vi "SubVI_Interpolate_Impedances.vi"(8 "error in (no error)":errorcluster, 9 "Resampling rate":dbl, 10 "Interpolant Size":dbl, 11 "Raw Impedances In":T1) -> (0 "error out":errorcluster, 3 "Interpolated Impedances Out":T2)   [LabVIEW 2020]
uses:
  <extravilib>/ChannelInstances/Stream-a[.](dbl)/)Channel.ctl
  <extravilib>/ChannelInstances/Lossy Stream-a[.](dbl)/)Channel.ctl
  <extravilib>/ChannelInstances/Lossy Stream-a[.](dbl)/EndpointRead.vi
  <extravilib>/ChannelInstances/Stream-a[.](dbl)/Endpoint.vi
  Global 1.vi
  <extravilib>/ChannelInstances/Lossy Stream-a[.](dbl)/)Channel.vi
  <resource>/ChannelSupport/_ChannelSupport/WaitIfNeeded.vi
  <extravilib>/ChannelInstances/Stream-a[.](dbl)/)Channel.vi
  <vilib>/ptbypt/NI_PtbyPt.lvlib
  <extravilib>/ChannelInstances/Stream-a[.](dbl).lvlib
  <extravilib>/ChannelInstances/Lossy Stream-a[.](dbl).lvlib
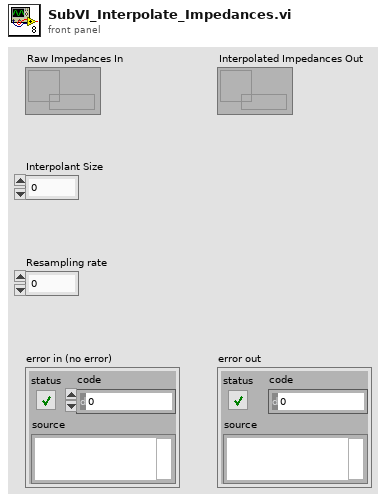
[diagram p1: front panel]
types:
  T1 = typedef "Lossy Stream-a[.](dbl).lvlib/)Channel.ctl" = refnum<queue>
  T2 = typedef "Stream-a[.](dbl).lvlib/)Channel.ctl" = refnum<queue>
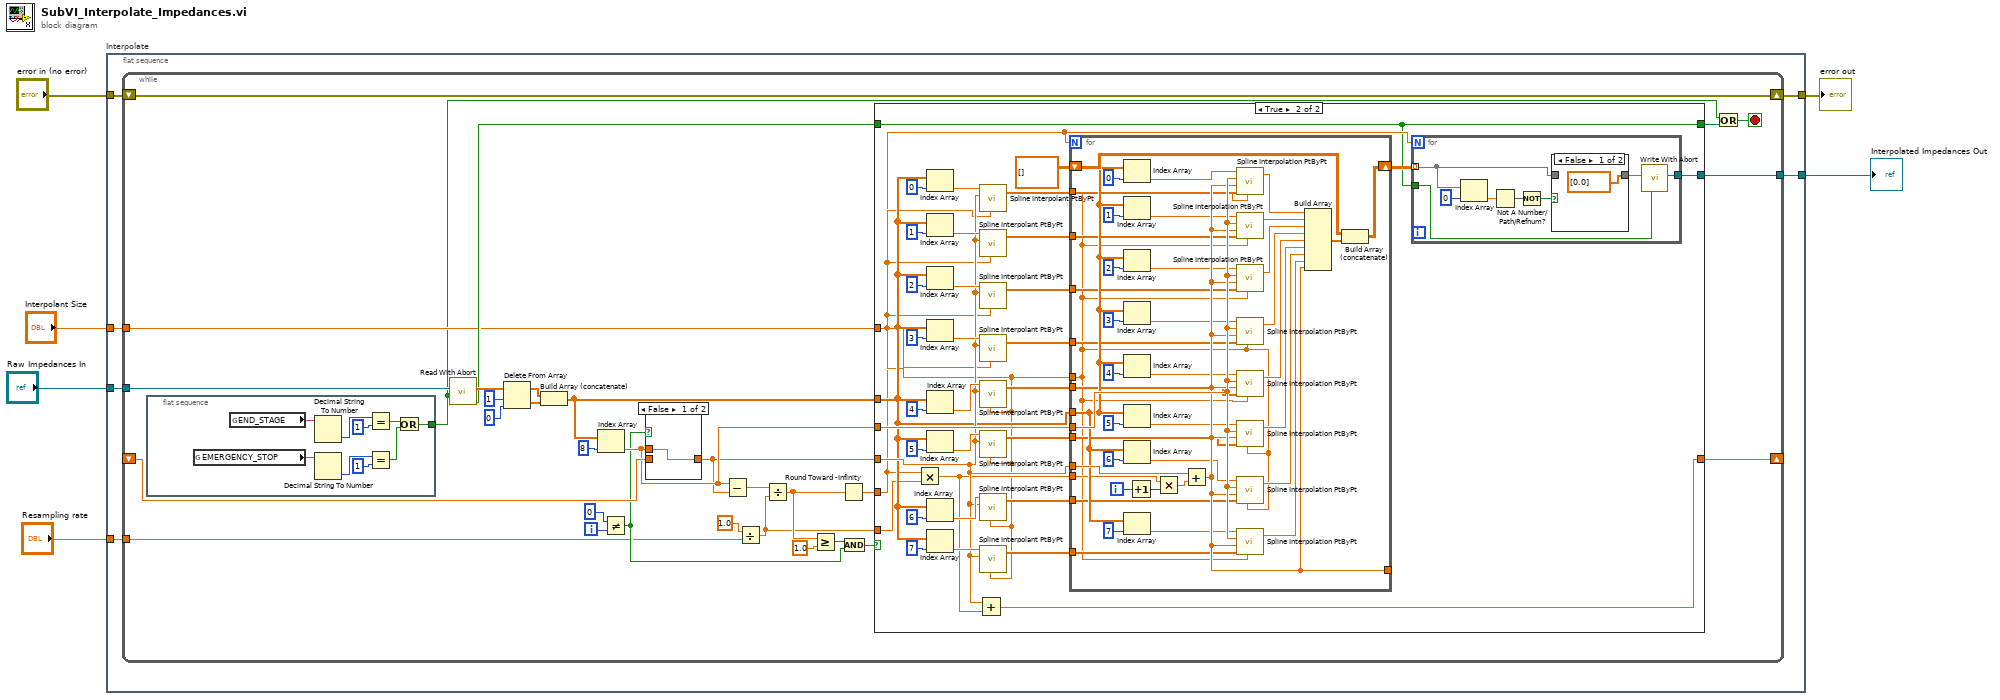
[diagram p0: block diagram]
diagram:
  n1 = flat-sequence "Interpolate" {
    tunnel: "Raw Impedances In" -> [w12]
    tunnel: [w11] -> w2
    tunnel: [w10] -> w3
    tunnel: "Interpolant Size" -> [w9]
    tunnel: "error in (no error)" -> [w8]
    tunnel: "Resampling rate" -> [w7]
    frame #0 {
      n2 = while {
        tunnel: w12 -> [w43]
        shift-right: [w26] -> _
        shift-left: _ -> [w31]
        shift-right: [w23] -> w11
        shift-left: w8 -> [w23]
        tunnel: w9 -> [w18]
        tunnel: [w17] -> w10
        tunnel: w7 -> [w16]
        i -> [w19]
        stop <- w21 stop-if-true
        n3 = flat-sequence {
          tunnel: [w44] -> w13
          frame #0 {
            n4 = global read "Global 1.vi" "EMERGENCY_STOP"() -> (w47:string)
            n5 = global read "Global 1.vi" "END_STAGE"() -> (w52:string)
            n6 = Decimal String To Number(string=w52) -> (number=w51:i32)  [unwired: 2 in, 1 out]
            n7 = Decimal String To Number(string=w47) -> (number=w49:i32)  [unwired: 2 in, 1 out]
            n8 = Equal?(x=w51, y=1) -> (x = y?=w45:bool)
            n9 = Equal?(x=w49, y=1) -> (x = y?=w46:bool)
            n10 = Or(x=w45, y=w46) -> (x .or. y?=w44:bool)
          }
        }
        n11 = call <extravilib>:"Read With Abort.vi"("abort"=w13, "channel"=w43) -> ("element"=w42:dbl[], "aborted?"=w27:bool)  [unwired: 3 in, 5 out]
        n12 = Delete From Array(array=w42, length=1, index=0) -> (deleted portion=w39:dbl[], array with subset deleted=w20:dbl[])
        n13 = Build Array (concatenate)(w20, w39) -> (w24:dbl[])
        n14 = Index Array(array=w24, index=8 ("disabled index (col)")) -> (element=w30:dbl)
        n15 = Not Equal?(x=0, y=w19) -> (x != y?=w25:bool)
        n16 = case shown="False" w25 {
          tunnel: w31 -> [_ w54]
          tunnel: [w53 w54] -> w28
          tunnel: w30 -> [w53 _]
          frame False {
          }
          frame True {
          }
        }
        n17 = Subtract(x=w30, y=w28) -> (x-y=w35:dbl)
        n18 = Divide(x=1.0 ("Resampling rate"), y=w16) -> (x/y=w14:dbl)
        n19 = Divide(x=w35, y=w14) -> (x/y=w33:dbl)
        n20 = Greater Or Equal?(x=w33, y=1.0) -> (x >= y?=w37:bool)
        n21 = Round Toward -Infinity(1:w33) -> (0:w29:dbl)
        n22 = And(x=w37, y=w25) -> (x .and. y?=w32:bool)
        n23 = case shown="True" w32 {
          tunnel: w30 -> [_ w92]
          tunnel: w28 -> [w56 w66]
          tunnel: [w56 w61] -> w26
          tunnel: w27 -> [w55 w57]
          tunnel: w29 -> [_ w59]
          tunnel: w24 -> [_ w65]
          tunnel: [w55 w57] -> w22
          tunnel: w14 -> [_ w64]
          tunnel: w18 -> [_ w62]
          tunnel: [_ w58] -> w17
          frame False {
          }
          frame True {
            n24 = Multiply(x=w59, y=w64) -> (x*y=w63:dbl)
            n25 = Index Array(array=w65, index=0) -> (element=w67:dbl)
            n26 = Index Array(array=w65, index=1) -> (element=w68:dbl)
            n27 = Index Array(array=w65, index=2) -> (element=w69:dbl)
            n28 = Index Array(array=w65, index=3) -> (element=w70:dbl)
            n29 = Index Array(array=w65, index=4) -> (element=w71:dbl)
            n30 = Index Array(array=w65, index=5) -> (element=w72:dbl)
            n31 = Index Array(array=w65, index=6) -> (element=w73:dbl)
            n32 = Index Array(array=w65, index=7) -> (element=w74:dbl)
            n33 = Add(x=w66, y=w63) -> (x+y=w61:dbl)
            n34 = call <vilib>:"Spline Interpolant PtByPt.vi"("sample length"=w62, "x"=w66, "y"=w67) -> ("Interpolant"=w83:dbl[])  [unwired: 3 in, 1 out]
            n35 = call <vilib>:"Spline Interpolant PtByPt.vi"("sample length"=w62, "x"=w66, "y"=w68) -> ("Interpolant"=w84:dbl[])  [unwired: 3 in, 1 out]
            n36 = call <vilib>:"Spline Interpolant PtByPt.vi"("sample length"=w62, "x"=w66, "y"=w69) -> ("Interpolant"=w85:dbl[])  [unwired: 3 in, 1 out]
            n37 = call <vilib>:"Spline Interpolant PtByPt.vi"("sample length"=w62, "x"=w66, "y"=w70) -> ("Interpolant"=w86:dbl[])  [unwired: 3 in, 1 out]
            n38 = call <vilib>:"Spline Interpolant PtByPt.vi"("sample length"=w62, "x"=w66, "y"=w71) -> ("Interpolant"=w87:dbl[])  [unwired: 3 in, 1 out]
            n39 = call <vilib>:"Spline Interpolant PtByPt.vi"("sample length"=w62, "x"=w66, "y"=w72) -> ("Interpolant"=w88:dbl[])  [unwired: 3 in, 1 out]
            n40 = call <vilib>:"Spline Interpolant PtByPt.vi"("sample length"=w62, "x"=w66, "y"=w73) -> ("Interpolant"=w89:dbl[])  [unwired: 3 in, 1 out]
            n41 = call <vilib>:"Spline Interpolant PtByPt.vi"("sample length"=w62, "x"=w66, "y"=w74) -> ("Interpolant"=w90:dbl[])  [unwired: 3 in, 1 out]
            n42 = for {
              N: w59 -> [_]
              tunnel: w83 -> [w112]
              tunnel: w84 -> [w111]
              tunnel: w85 -> [w110]
              tunnel: w86 -> [w109]
              tunnel: w87 -> [w108]
              tunnel: w88 -> [w107]
              tunnel: w89 -> [w106]
              tunnel: w90 -> [w105]
              tunnel: w92 -> [w139]
              tunnel: w66 -> [w138]
              tunnel: [w137] -> _
              shift-right: [w134] -> w60
              shift-left: dbl[][] [] -> [w133]
              tunnel: w65 -> [w113]
              tunnel: w63 -> [w104]
              tunnel: w62 -> [w103]
              i -> [w116]
              n43 = Index Array(array=w113, index=0) -> (element=w124:dbl)
              n44 = Index Array(array=w113, index=1) -> (element=w123:dbl)
              n45 = Index Array(array=w113, index=2) -> (element=w122:dbl)
              n46 = Index Array(array=w113, index=3) -> (element=w121:dbl)
              n47 = Index Array(array=w113, index=4) -> (element=w120:dbl)
              n48 = Index Array(array=w113, index=5) -> (element=w119:dbl)
              n49 = Index Array(array=w113, index=6) -> (element=w118:dbl)
              n50 = Index Array(array=w113, index=7) -> (element=w117:dbl)
              n51 = Increment(x=w116) -> (x+1=w115:i32)
              n52 = Multiply(x=w104, y=w115) -> (x*y=w135:dbl)
              n53 = Add(x=w138, y=w135) -> (x+y=w137:dbl)
              n54 = call <vilib>:"Spline Interpolation PtByPt.vi"("sample length"=w103, "Interpolant"=w112, "x value"=w137, "x"=w139, "y"=w124) -> ("interpolation value"=w136:dbl)  [unwired: 1 in, 1 out]
              n55 = call <vilib>:"Spline Interpolation PtByPt.vi"("sample length"=w103, "Interpolant"=w111, "x value"=w137, "x"=w139, "y"=w123) -> ("interpolation value"=w146:dbl)  [unwired: 1 in, 1 out]
              n56 = call <vilib>:"Spline Interpolation PtByPt.vi"("sample length"=w103, "Interpolant"=w110, "x value"=w137, "x"=w139, "y"=w122) -> ("interpolation value"=w145:dbl)  [unwired: 1 in, 1 out]
              n57 = call <vilib>:"Spline Interpolation PtByPt.vi"("sample length"=w103, "Interpolant"=w109, "x value"=w137, "x"=w139, "y"=w121) -> ("interpolation value"=w144:dbl)  [unwired: 1 in, 1 out]
              n58 = call <vilib>:"Spline Interpolation PtByPt.vi"("sample length"=w103, "Interpolant"=w108, "x value"=w137, "x"=w139, "y"=w120) -> ("interpolation value"=w143:dbl)  [unwired: 1 in, 1 out]
              n59 = call <vilib>:"Spline Interpolation PtByPt.vi"("sample length"=w103, "Interpolant"=w107, "x value"=w137, "x"=w139, "y"=w119) -> ("interpolation value"=w142:dbl)  [unwired: 1 in, 1 out]
              n60 = call <vilib>:"Spline Interpolation PtByPt.vi"("sample length"=w103, "Interpolant"=w106, "x value"=w137, "x"=w139, "y"=w118) -> ("interpolation value"=w141:dbl)  [unwired: 1 in, 1 out]
              n61 = call <vilib>:"Spline Interpolation PtByPt.vi"("sample length"=w103, "Interpolant"=w105, "x value"=w137, "x"=w139, "y"=w117) -> ("interpolation value"=w140:dbl)  [unwired: 1 in, 1 out]
              n62 = Build Array(w136, w146, w145, w144, w143, w142, w141, w140, w137) -> (w114:dbl[])
              n63 = Build Array (concatenate)(w133, w114) -> (w134:dbl[][])
            }
            n64 = for {
              N: w59 -> [_]
              tunnel: w60 -> [w94] mode=indexing
              tunnel: w57 -> [w96]
              tunnel: [w95] -> w58
              n65 = Index Array(array=w94, index=0) -> (element=w99:dbl)
              n66 = Not A Number/Path/Refnum?(number/path/refnum=w99) -> (NaN/Path/Refnum?=w98:bool)
              n67 = Not(x=w98) -> (.not. x?=w97:bool)
              n68 = case shown="False" w97 {
                tunnel: w94 -> [_ w102]
                tunnel: [dbl[] [0.0] w102] -> w93
                frame False {
                }
                frame True {
                }
              }
              n69 = call <extravilib>:"Write With Abort.vi"("abort"=w96, "element"=w93) -> ("channel"=w95:T2)  [unwired: 6 in, 3 out]
            }
          }
        }
        n70 = Or(x=w13, y=w22) -> (x .or. y?=w21:bool)
      }
    }
  }
  "Interpolated Impedances Out" <- w3
  "error out" <- w2
